vi "平行样测试全局变量.vi"() -> ()   [LabVIEW 2016, in "质控单元.lvlib"]
panel:
  in  "CODcr":T1={"时间标识"=timestamp(0 s since 1904-01-01), "参数"="CODCr平行样测试", "第一次水样浓度值"=0.0, "第二次水样测试时间"=timestamp(0 s since 1904-01-01), "第二次水样浓度值"=0.0}
  in  "CODMn":T1={"时间标识"=timestamp(0 s since 1904-01-01), "参数"="CODMn平行样测试", "第一次水样浓度值"=0.0, "第二次水样测试时间"=timestamp(0 s since 1904-01-01), "第二次水样浓度值"=0.0}
  in  "总氮":T1={"时间标识"=timestamp(0 s since 1904-01-01), "参数"="总氮平行样测试", "第一次水样浓度值"=0.0, "第二次水样测试时间"=timestamp(0 s since 1904-01-01), "第二次水样浓度值"=0.0}
  in  "总磷":T1={"时间标识"=timestamp(0 s since 1904-01-01), "参数"="总磷平行样测试", "第一次水样浓度值"=0.0, "第二次水样测试时间"=timestamp(0 s since 1904-01-01), "第二次水样浓度值"=0.0}
  in  "氨氮":T1={"时间标识"=timestamp(0 s since 1904-01-01), "参数"="氨氮平行样测试", "第一次水样浓度值"=0.0, "第二次水样测试时间"=timestamp(0 s since 1904-01-01), "第二次水样浓度值"=0.0}
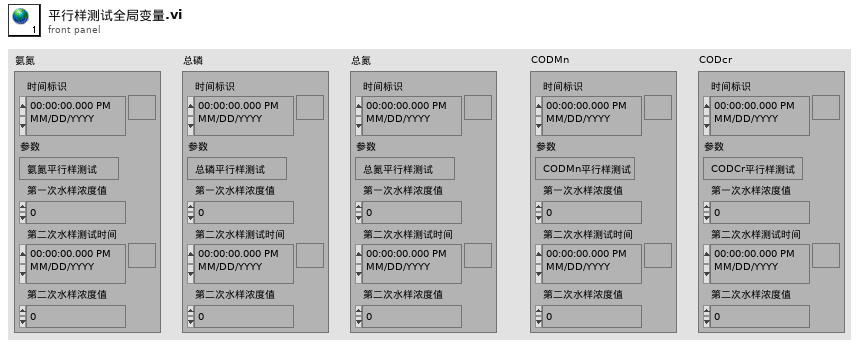
[diagram p1: front panel]
types:
  T1 = cluster{"时间标识":timestamp, "参数":string, "第一次水样浓度值":sgl, "第二次水样测试时间":timestamp, "第二次水样浓度值":sgl}
diagram:
